vi "API_GetVersion.vi"() -> (2 "Version":sgl, 3 "Windows NT":bool)   [LabVIEW 2011, in "API.lvlib"]
uses:
  API.lvlib
  kernel32.dll
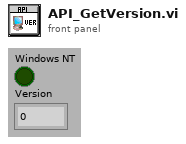
[diagram p1: front panel]
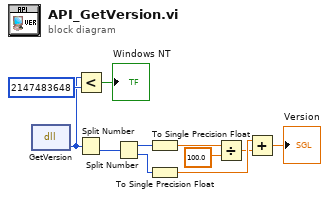
[diagram p0: block diagram]
diagram:
  n1 = dll-call lib="kernel32.dll" fn="GetVersion"() -> ("Versions"=w2:u32)  [unwired: 3 in, 2 out]
  n2 = Less?(x=w2, y=u32 2147483648) -> (x < y?=→"Windows NT":bool)
  n3 = Split Number(x=w2) -> (lo(x)=w9:u16)  [unwired: 1 out]
  n4 = Split Number(x=w9) -> (hi(x)=w4:u8, lo(x)=w3:u8)
  n5 = To Single Precision Float(number=w4) -> (single precision float=w5:sgl)
  n6 = To Single Precision Float(number=w3) -> (single precision float=w8:sgl)
  n7 = Divide(x=w5, y=sgl 100.0) -> (x/y=w7:sgl)
  n8 = Add(x=w8, y=w7) -> (x+y=→"Version":sgl)
